vi "Discover Plugins from Loader.vi"(8 "error in (no error)":errorcluster, 10 "Discovery Command":T1, 11 "CIFPluginManager in":refnum<class "CIFPluginManager.lvclass">) -> (0 "error out":errorcluster)   [LabVIEW 2021, in "CIFPluginManager.lvclass"]
uses:
  CIFPluginManager.lvclass
  typedef/Discover Command.ctl
  CIFPluginManager.lvclass/CIFPluginManager.ctl
  typedef/Discovered Plugin.ctl
  <vilib>/CIF Foundation/CIF Core/CIFCore/Common/Typedef/Version.ctl
  typedef/Plugin Metadata.ctl
  typedef/Loader Type.ctl
  <vilib>/CIF Foundation/CIF Core/CIFCore/Common/Typedef/Errors.ctl
  <vilib>/CIF Foundation/CIF Utilities/Errors/Append Error Location.vi
  <vilib>/CIF Foundation/CIF Core/CIFCore/Common/CIFCoreCommon.lvlib
  CIFPluginLoader/gRPC/CIF_Plugin_Loader_Client_Wrapper/CIFPluginLoaderClientWrapper.lvlib
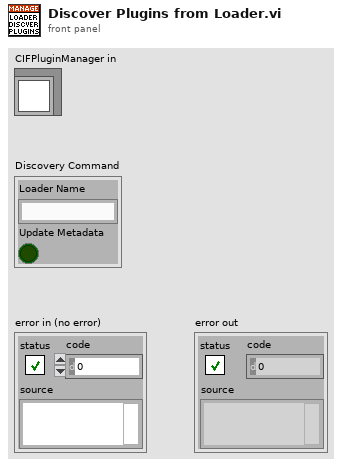
[diagram p1: front panel]
types:
  T1 = typedef "CIFPluginManager.lvclass/Discover Command.ctl" = cluster{"Loader Name":string, "Update Metadata":bool}
  T2 = typedef "CIFPluginManager.lvclass/Loader Map.ctl" = map{string, T3}
  T3 = typedef "CIFPluginManager.lvclass/Loaders.ctl" = cluster{"Loader Type":T4, "grpc_port":i32, "pid":u32, "gRPC ID":T5, "Load Timestamp":i64, "Unloading":bool, "Ready for removal":bool, "Unload Timestamp":i64}
  T4 = typedef "CIFPluginManager.lvclass/Loader Type.ctl" = enum16{"LabVIEW"}
  T5 = typedef "grpc-lvsupport-release.lvlib/grpcId.ctl" = u64
  T6 = typedef "CIFPluginManager.lvclass/Discovered Plugin.ctl" = cluster{"Filename":string, "Plugin Type":string, "Qualified name":string, "Version":T7, "Plugin Metadata":T8, "Loader Type":T4, "File Path":string, "Relative Path":string[]}
  T7 = typedef "CIFCoreCommon.lvlib/Version.ctl" = cluster{"Major":i32, "Minor":i32, "Fix":i32, "Build":i32}
  T8 = typedef "CIFPluginManager.lvclass/Plugin Metadata.ctl" = cluster{"Description":string, "History":string, "Author":string}
  T9 = typedef "CIF_PluginLoader_client.lvlib/cif_pluginloader_DiscoveredPlugin.ctl" = cluster{"file_path":string, "file_name":string, "plugin_type":string, "plugin_version":T10, "plugin_metadata":T11, "relative_path":string[]}
  T10 = typedef "CIF_PluginLoader_client.lvlib/cif_common_Version.ctl" = cluster{"major":u32, "minor":u32, "fix":u32, "build":u32}
  T11 = typedef "CIF_PluginLoader_client.lvlib/cif_management_common_PluginMetadata.ctl" = cluster{"description":string, "history":string, "author":string}
  T12 = typedef "CIFPluginManager.lvclass/Discovered Plugin Map.ctl" = map{string, T6[]}
  T13 = typedef "CIFCoreCommon.lvlib/Errors.ctl" = enum16{"Invalid Clock ID", "Long Sleep", "gRPC Server Not Found", "Config Parse", "Timestamp Wrap", "Delayed Execution", "Duplicate Channel", "Missing Channel", "Incorrect Type", "Flatten Error", "Unflatten Data", "Unique Name", "Plugin Not Found", "Plugin Type Not Found", "Plugin Version Not Found", "Manager Not Found", "Numerical Issue", "Time Jump", "Clock ID Match", "Channel Length", "Plugin Connection", "gRPC Server Connection", "PPL Name Match", "Build", "Config Log Parse", "Plugin Load", "UI Subpanel Load", "Python Name", "Invalid Name", "Unable to Change Ch Buffer", "Failed Kill", "Failed SysExec", "Function Not Implemented", "Load Timeout"}
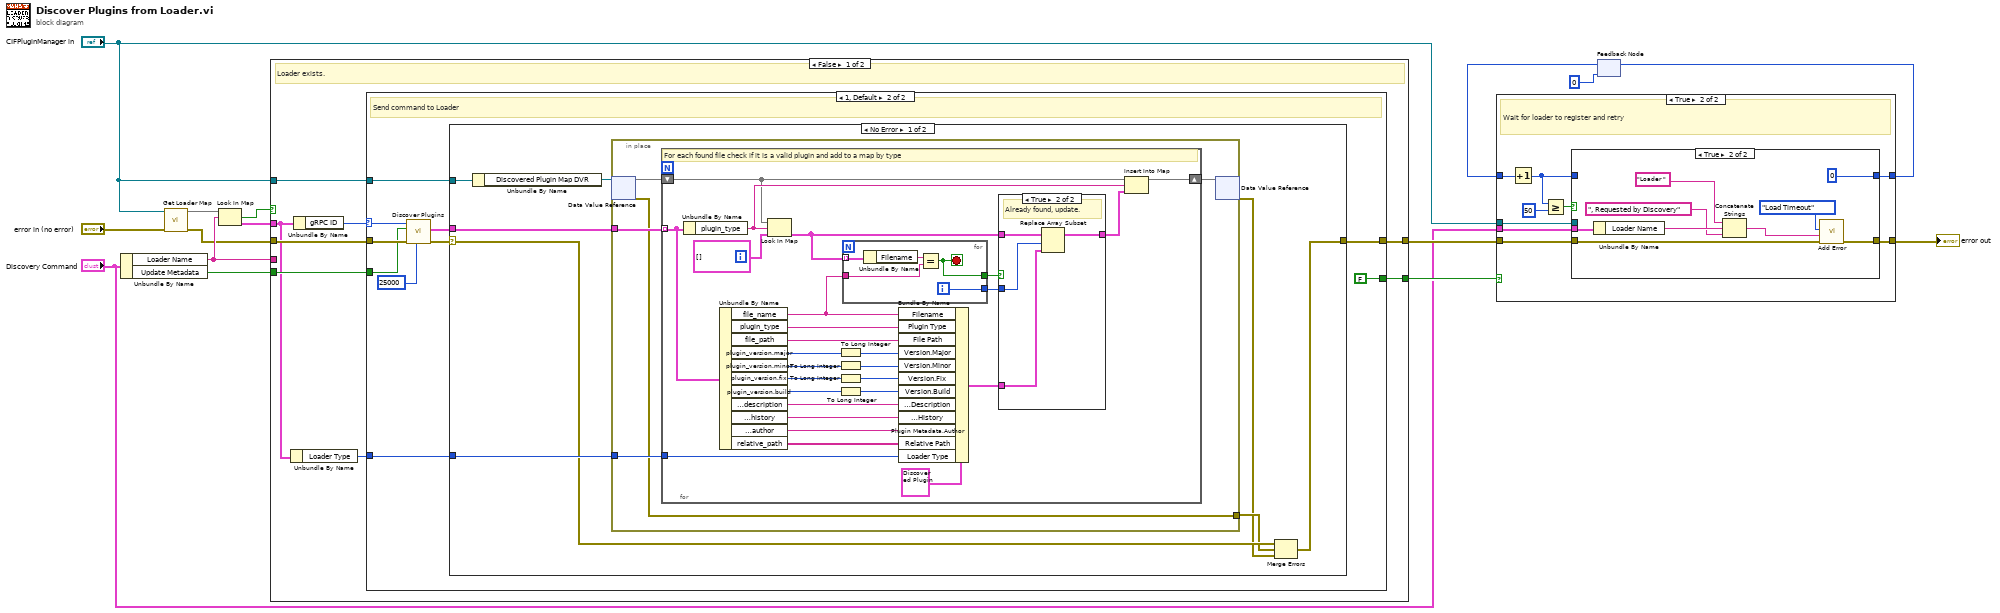
[diagram p0: block diagram]
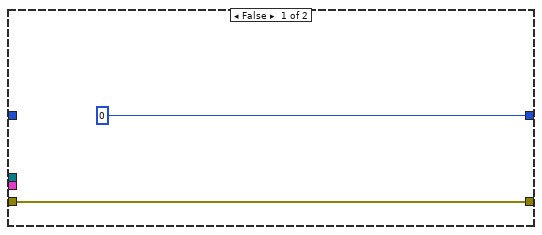
[diagram p2: hidden frame]
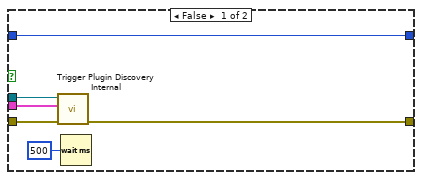
[diagram p3: hidden frame]
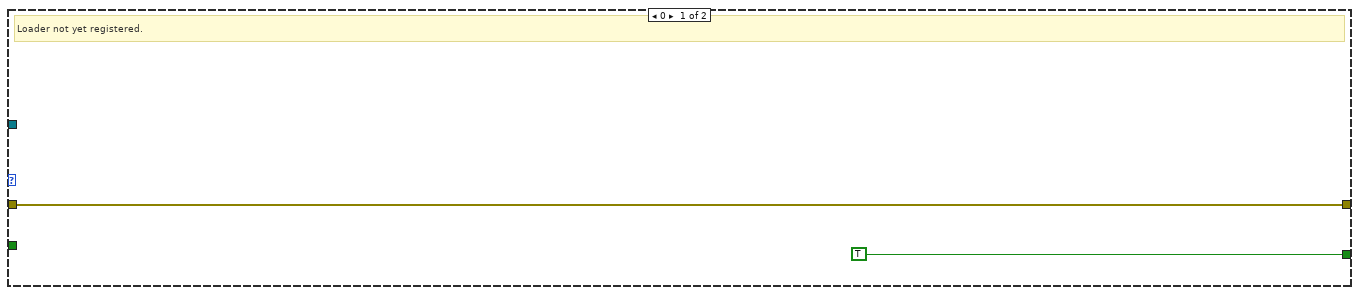
[diagram p4: hidden frame]
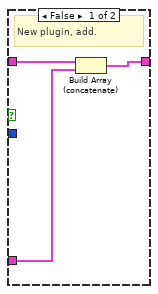
[diagram p5: hidden frame]
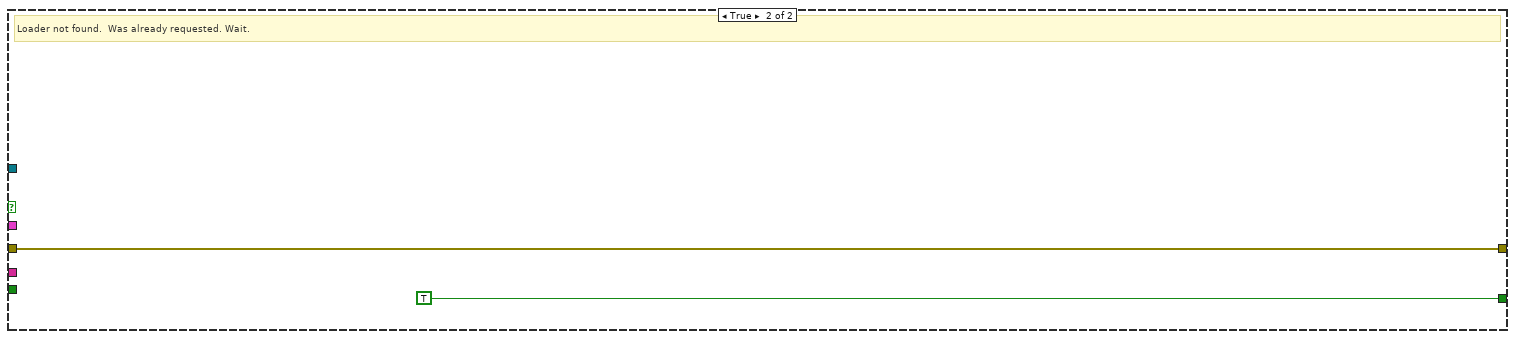
[diagram p7: hidden frame]
diagram:
  n1 = Unbundle By Name("Discovery Command") -> ("Loader Name"=w11:string, "Update Metadata"=w9:bool)
  n2 = call "Get Loader Map.vi"("error in (no error)"="error in (no error)", "CIFPluginManager in"="CIFPluginManager in") -> ("error out"=w6:errorcluster, "Loader Map"=w7:T2)  [unwired: 8 in]
  n3 = Look In Map(map=w7, key=w11) -> (key not found?=w15:bool, value=w13:T3)  [unwired: 1 in]
  n4 = case shown="False" w15 {
    tunnel: "CIFPluginManager in" -> [w19 _]
    tunnel: w6 -> [w20 w89]
    tunnel: [w21 w89] -> w12
    tunnel: w11 -> [_ _]
    tunnel: [w22 TRUE] -> w14
    tunnel: w13 -> [w17 _]
    tunnel: w9 -> [w18 _]
    frame False {
      # "Loader exists."
      n5 = Unbundle By Name(w17) -> ("Loader Type"=w16:T4)
      n6 = Unbundle By Name(w17) -> ("gRPC ID"=w23:T5)
      n7 = case shown="1, Default" w23 {
        selector: w23 -> [_ w35]
        tunnel: [TRUE FALSE] -> w22
        tunnel: [w24 w32] -> w21
        tunnel: w20 -> [w24 w34]
        tunnel: w19 -> [_ w28]
        tunnel: w18 -> [_ w30]
        tunnel: w16 -> [_ w27]
        frame 0 {
          # "Loader not yet registered."
        }
        frame 1, Default {
          # "Send command to Loader"
          n8 = call "Discover Plugins.vi"("timeout (ms)"=25000, "error in"=w34, "update_metadata"=w30, "gRPC ID in"=w35) -> ("error out"=w31:errorcluster, "discovered_plugins"=w29:T9[])  [unwired: 5 in, 1 out]
          n9 = case shown="No Error" w31 {
            selector: w31 -> [w39 w88]
            tunnel: [w36 w88] -> w32
            tunnel: w29 -> [w42 _]
            tunnel: w28 -> [w43 _]
            tunnel: w27 -> [w41 _]
            frame No Error {
              n10 = Unbundle By Name(w43) -> ("Discovered Plugin Map DVR"=w40:refnum<data-value>)
              n11 = in-place {
                in-place-border: w42 -> [w48]
                in-place-border: w41 -> [w47]
                in-place-border: [w44] -> w38
                n12 = in-place-dvr #1(w40) -> (w46:T12, w44:errorcluster)
                n13 = for {
                  tunnel: w48 -> [w65] mode=indexing
                  shift-right: [w68] -> w45
                  shift-left: w46 -> [w69]
                  tunnel: w47 -> [w50]
                  # "For each found file check if it is a valid plugin and add to a map by type"
                  n14 = Unbundle By Name(w65) -> ("plugin_type"=w70:string)
                  n15 = Unbundle By Name(w65) -> ("file_name"=w64:string, "plugin_type"=w63:string, "file_path"=w62:string, "plugin_version.major"=w51:u32, "plugin_version.minor"=w52:u32, "plugin_version.fix"=w61:u32, "plugin_version.build"=w60:u32, "plugin_metadata.description"=w55:string, "plugin_metadata.history"=w54:string, "plugin_metadata.author"=w53:string, "relative_path"=w49:string[])
                  n16 = Look In Map(map=w69, key=w70, default value=T6[] [] ("value")) -> (value=w73:T6[])  [unwired: 1 out]
                  n17 = To Long Integer(number=w51) -> (32bit integer=w59:i32)
                  n18 = To Long Integer(number=w52) -> (32bit integer=w58:i32)
                  n19 = To Long Integer(number=w61) -> (32bit integer=w57:i32)
                  n20 = To Long Integer(number=w60) -> (32bit integer=w56:i32)
                  n21 = for {
                    tunnel: w64 -> [w86]
                    tunnel: w73 -> [w83] mode=indexing
                    tunnel: [w85] -> w74
                    tunnel: [w84] -> w72
                    i -> [w84]
                    stop <- w85 stop-if-true
                    n22 = Unbundle By Name(w83) -> ("Filename"=w87:string)
                    n23 = Equal?(x=w87, y=w86) -> (x = y?=w85:bool)
                  }
                  n24 = Bundle By Name(cluster=T6 {"Filename"="", "Plugin Type"="", "Qualified name"="", "Version"={"Major"=0, "Minor"=0, "Fix"=0, "Build"=0}, "Plugin Metadata"={"Description"="", "History"="", "Author"=""}, "Loader Type"=enum."LabVIEW", "File Path"="", "Relative Path"=[]} ("Discovered Plugin"), "Filename"=w64, "Plugin Type"=w63, "File Path"=w62, "Version.Major"=w59, "Version.Minor"=w58, "Version.Fix"=w57, "Version.Build"=w56, "Plugin Metadata.Description"=w55, "Plugin Metadata.History"=w54, "Plugin Metadata.Author"=w53, "Relative Path"=w49, "Loader Type"=w50) -> (w67:T6)
                  n25 = case shown="True" w74 {
                    tunnel: w67 -> [w77 w82]
                    tunnel: w73 -> [w78 w81]
                    tunnel: [w76 w79] -> w71
                    tunnel: w72 -> [_ w80]
                    frame False {
                      # "New plugin, add."
                      n26 = Build Array (concatenate)(w78, w77) -> (w76:T6[])
                    }
                    frame True {
                      # "Already found, update."
                      n27 = Replace Array Subset(array=w81, new element=w82, index=w80) -> (w79:T6[])
                    }
                  }
                  n28 = Insert Into Map(map in=w69, key=w70, value=w71) -> (map out=w68:T12)  [unwired: 2 out]
                }
                n29 = in-place-dvr #1(w45) -> (w37:errorcluster)  [unwired: 1 out]
              }
              n30 = Merge Errors(w39, w38, w37) -> (w36:errorcluster)
            }
            frame Error {
            }
          }
        }
      }
    }
    frame True {
      # "Loader not found.  Was already requested. Wait."
    }
  }
  n31 = feedback #2(0) -> (w2:i32)
  n32 = case shown="True" w14 {
    tunnel: w12 -> [w92 w99]
    tunnel: "CIFPluginManager in" -> [_ w101]
    tunnel: "Discovery Command" -> [_ w100]
    tunnel: [w92 w98] -> w5
    tunnel: w2 -> [_ w97]
    tunnel: [0 w93] -> w1
    frame False {
    }
    frame True {
      # "Wait for loader to register and retry"
      n33 = Increment(x=w97) -> (x+1=w94:i32)
      n34 = Greater Or Equal?(x=w94, y=50) -> (x >= y?=w96:bool)
      n35 = case shown="True" w96 {
        tunnel: w101 -> [w106 _]
        tunnel: w100 -> [w105 w112]
        tunnel: w99 -> [w104 w116]
        tunnel: [w103 w115] -> w98
        tunnel: w94 -> [w102 _]
        tunnel: [w102 0] -> w93
        frame False {
          n36 = call "Trigger Plugin Discovery Internal.vi"("error in (no error)"=w104, "Trigger Discovery"=w105, "CIFPluginManager in"=w106) -> ("error out"=w103:errorcluster)  [unwired: 8 in]
          n37 = Wait (ms)(milliseconds to wait=u32 500) -> ()  [unwired: 1 out]
        }
        frame True {
          n38 = Unbundle By Name(w112) -> ("Loader Name"=w110:string)
          n39 = Concatenate Strings("Loader " ("String to Append"), w110, ", Requested by Discovery" ("string")) -> (w108:string)
          n40 = call <vilib>:"Add Error.vi"("error in (no error)"=w116, "String to Append"=w108, "Error"=Errors."Load Timeout") -> ("error out"=w115:errorcluster)  [unwired: 8 in]
        }
      }
    }
  }
  "error out" <- w5
  n41 = feedback-in #2(w1) -> ()
